vi "ArmLoop2.vi"(11 "ArmRef":T2={"Pot"={"DevStatus"={"status"=FALSE, "code"=0, "source"=""}, "Analog Channel"=enum."Invalid", "Invert Output"=FALSE}, "ArmMotor"={"DeviceStatus"={"status"=FALSE, "code"=0, "source"=""}, "Type"=enum."PWM", "PWM"={"PWM Channel"=enum."Invalid", "DeadBand"={"Name"="", "maxPositivePwm"=0, "minPositivePwm"=0, "centerPwm"=0, "maxNegativePwm"=0, "minNegativePwm"=0, "angularRange"=0}}, "CAN"={"Device Number"=0, "Control Mode"=enum."Percent VBus", "Semaphore"=refnum, "Max Vout"=12.0, "TalonSRX Control Mode"=enum."Percent VBus"}, "Invert"=FALSE}, "Queue"=refnum, "Setpoint"=0.0, "Manual"=FALSE, "output range"={"output high"=100.0, "output low"=-0.38}, "PID gains"={"proportional gain (Kc)"=1.0, "integral time (Ti, min)"=0.01, "derivative time (Td, min)"=0.0}}) -> ()   [LabVIEW 2015, in "ArmController.lvlib"]
uses:
  ArmController.lvlib
  Typedef/ArmRef.ctl
  <vilib>/Rock Robotics/WPI/Potentiometer/WPI_PotentiometerDevRef.ctl
  <vilib>/Rock Robotics/SystemInterfaces/AI/FPGA_AIChannel.ctl
  <vilib>/Rock Robotics/WPI/MotorControl/WPI_MotorControlDeviceRef.ctl
  <vilib>/Rock Robotics/WPI/MotorControl/WPI_MotorControlType.ctl
  <vilib>/Rock Robotics/SystemInterfaces/DIO/FPGA_DIOPWMChannel.ctl
  <vilib>/Rock Robotics/WPI/PWM/WPI_PWMDeadband.ctl
  <vilib>/Rock Robotics/WPI/CAN/Jaguar/SubVIs/WPI_CANJaguar_ControlMode.ctl
  <vilib>/Rock Robotics/WPI/CAN/TalonSRX/WPI_CANTalonSRX_APIControlMode.ctl
  Typedef/MessageType.ctl
  <vilib>/Rock Robotics/Network Tables/NT Write Number.vi
  <vilib>/addons/control/pid/pid.llb/PID Advanced (DBL).vi
  <vilib>/addons/control/pid/NI_PID_pid.lvlib
panel:
  out "Chart":T1(graph)
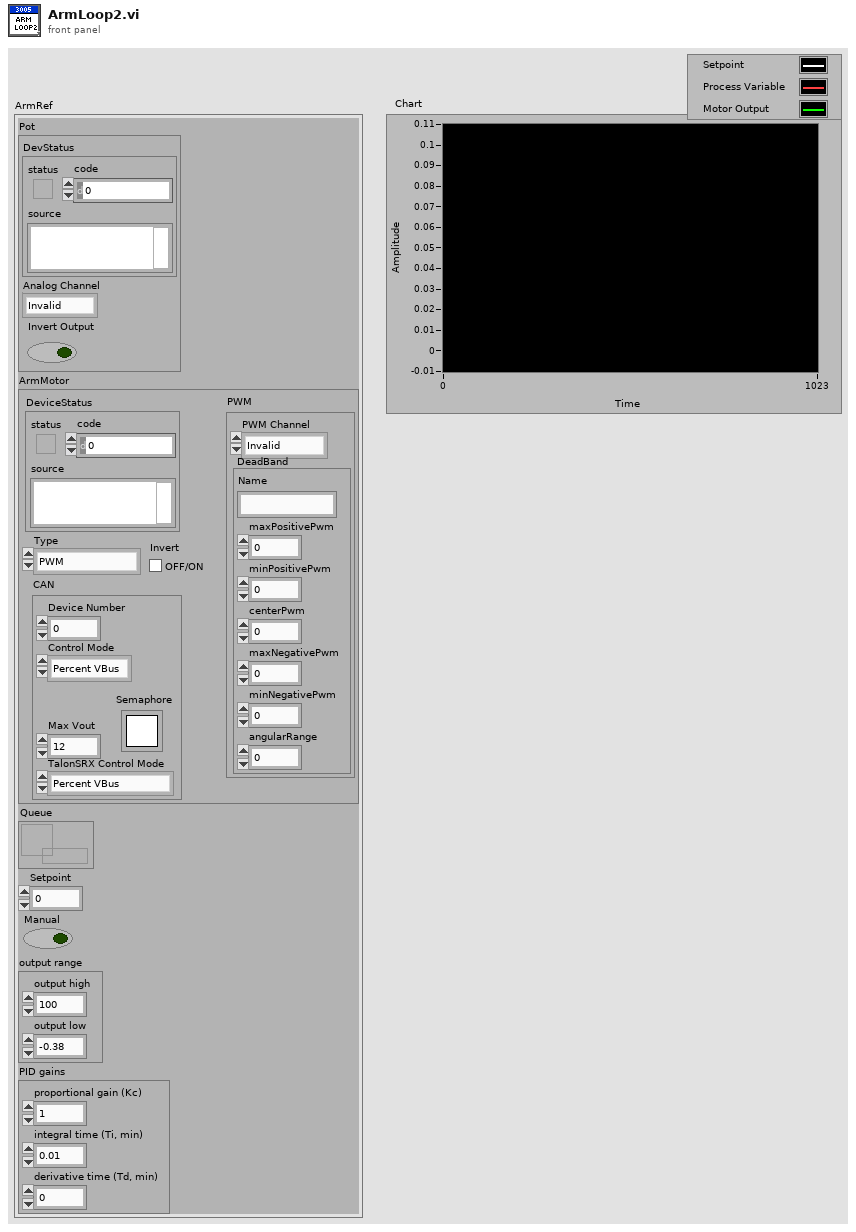
[diagram p1: front panel]
types:
  T1 = cluster{"Value":dbl, "Normalized Value":dbl, "output":dbl}
  T2 = typedef "ArmController.lvlib/ArmRef.ctl" = cluster{"Pot":T3, "ArmMotor":T5, "Queue":refnum<queue>, "Setpoint":dbl, "Manual":bool, "output range":cluster{"output high":dbl, "output low":dbl}, "PID gains":cluster{"proportional gain (Kc)":dbl, "integral time (Ti, min)":dbl, "derivative time (Td, min)":dbl}}
  T3 = typedef "WPI_PotentiometerDevRef.ctl" = cluster{"DevStatus":errorcluster, "Analog Channel":T4, "Invert Output":bool}
  T4 = typedef "FPGA_AIChannel.ctl" = enum8{"AI 0", "AI 1", "AI 2", "AI 3", "AI MXP 0", "AI MXP 1", "AI MXP 2", "AI MXP 3", "Invalid"}
  T5 = typedef "WPI_MotorControlDeviceRef.ctl" = cluster{"DeviceStatus":errorcluster, "Type":T6, "PWM":cluster{"PWM Channel":T7, "DeadBand":T8}, "CAN":cluster{"Device Number":u8, "Control Mode":T9, "Semaphore":T10, "Max Vout":dbl, "TalonSRX Control Mode":T11}, "Invert":bool}
  T6 = typedef "WPI_MotorControlType.ctl" = enum16{"PWM", "CAN", "CANTalonSRX"}
  T7 = typedef "FPGA_DIOPWMChannel.ctl" = enum8{"PWM 0", "PWM 1", "PWM 2", "PWM 3", "PWM 4", "PWM 5", "PWM 6", "PWM 7", "PWM 8", "PWM 9", "PWM MXP 0", "PWM MXP 1", "PWM MXP 2", "PWM MXP 3", "PWM MXP 4", "PWM MXP 5", "PWM MXP 6", "PWM MXP 7", "PWM MXP 8", "PWM MXP 9", "Invalid"}
  T8 = typedef "WPI_PWMDeadband.ctl" = cluster{"Name":string, "maxPositivePwm":i32, "minPositivePwm":i32, "centerPwm":i32, "maxNegativePwm":i32, "minNegativePwm":i32, "angularRange":u16}
  T9 = typedef "WPI_CANJaguar_ControlMode.ctl" = enum8{"Percent VBus", "Current", "Speed", "Position", "Voltage"}
  T10 = typedef "Semaphore RefNum" = refnum<k1>
  T11 = typedef "WPI_CANTalonSRX_APIControlMode.ctl" = enum8{"Percent VBus", "Speed", "Position", "Slave", "Unchanged / Invalid", "Voltage Compensation", "Current", "Motion Profile"}
  T12 = cluster{"proportional gain (Kc)":dbl, "integral time (Ti, min)":dbl, "derivative time (Td, min)":dbl}
  T13 = typedef "ArmController.lvlib/MessageType.ctl" = cluster{"Value":dbl, "Manual Control":bool, "Auto Switch":bool}
  T14 = cluster{"Setpoint":dbl, "Normalized Value":dbl, "output":dbl}
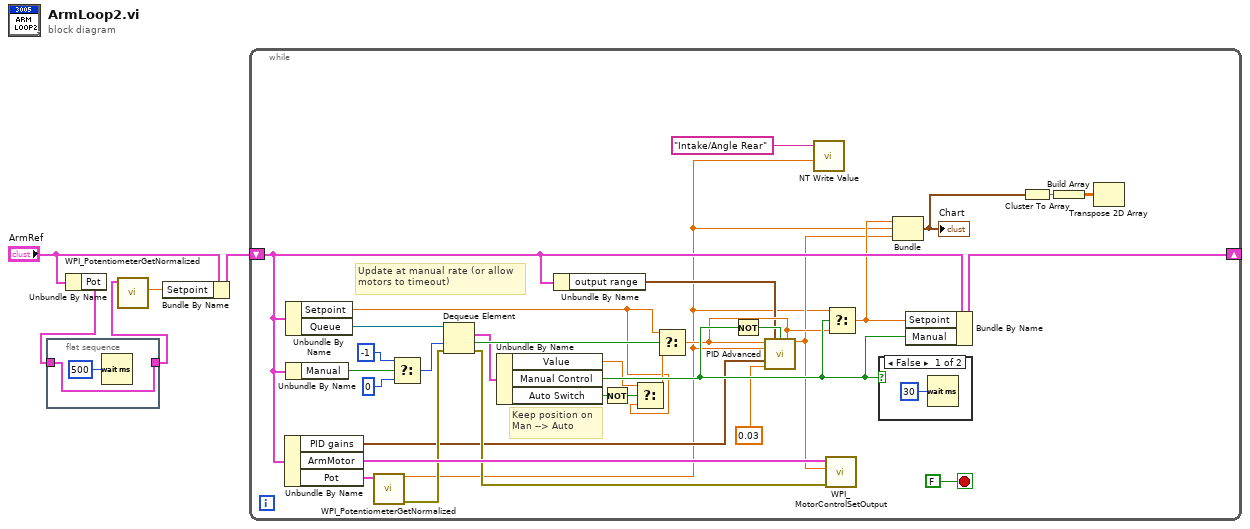
[diagram p0: block diagram]
diagram:
  n1 = flat-sequence {
    tunnel: w2 -> [w6]
    tunnel: [w6] -> w3
    frame #0 {
      n2 = Wait (ms)(milliseconds to wait=u32 500) -> ()  [unwired: 1 out]
    }
  }
  n3 = Unbundle By Name("ArmRef") -> ("Pot"=w2:T3)
  n4 = call <vilib>:"WPI_PotentiometerGetNormalized.vi"("PotDevRef"=w3) -> ("Normalized Value"=w5:dbl)  [unwired: 8 in, 2 out]
  n5 = Bundle By Name(cluster="ArmRef", "Setpoint"=w5) -> (w1:T2)
  n6 = while {
    shift-right: [w35] -> _
    shift-left: w1 -> [w23]
    stop <- FALSE stop-if-true
    # "Keep position on\nMan --> Auto"
    # "Update at manual rate (or allow\nmotors to timeout)"
    n7 = Unbundle By Name(w23) -> ("PID gains"=w18:T12, "ArmMotor"=w34:T5, "Pot"=w36:T3)
    n8 = Unbundle By Name(w23) -> ("Setpoint"=w13:dbl, "Queue"=w39:refnum<queue>)
    n9 = Unbundle By Name(w23) -> ("Manual"=w30:bool)
    n10 = call <vilib>:"WPI_PotentiometerGetNormalized.vi"("PotDevRef"=w36) -> ("error out"=w29:errorcluster, "Normalized Value"=w12:dbl)  [unwired: 8 in, 1 out]
    n11 = Select(t=-1 ("timeout in ms (-1)"), s=w30, f=0 ("timeout in ms (-1)")) -> (s? t:f=w31:i32)
    n12 = Dequeue Element(queue=w39, timeout in ms (-1)=w31, error in (no error)=w29) -> (element=w37:T13, timed out?=w38:bool, error out=w28:errorcluster)  [unwired: 1 out]
    n13 = Unbundle By Name(w37) -> ("Value"=w15:dbl, "Manual Control"=w27:bool, "Auto Switch"=w17:bool)
    n14 = Unbundle By Name(w23) -> ("output range"=w19:cluster{"output high":dbl, "output low":dbl})
    n15 = Not(x=w17) -> (.not. x?=w14:bool)
    n16 = Select(t=w15, s=w14, f=w13) -> (s? t:f=w16:dbl)
    n17 = Select(t=w13, s=w38, f=w16) -> (s? t:f=w26:dbl)
    n18 = Not(x=w27) -> (.not. x?=w20:bool)
    n19 = call-poly <vilib>:"PID Advanced.vi"("setpoint"=w26, "output range"=w19, "auto? (T)"=w20, "manual control"=w26, "process variable"=w12, "PID gains"=w18, "dt (s)"=0.03) -> ("output"=w21:dbl)  [unwired: 7 in, 1 out]
    n20 = call-poly <vilib>:"NT Write Value.vi"("Numeric"=w12, "Name"="Intake/Angle Rear") -> ()  [unwired: 9 in, 1 out]
    n21 = call <vilib>:"WPI_MotorControlSetOutput.vi"("error in (no error)"=w28, "Output"=w21, "MotorControlDevRef"=w34) -> ()  [unwired: 6 in, 3 out]
    n22 = Select(t=w12, s=w27, f=w26) -> (s? t:f=w22:dbl)
    n23 = case shown="False" w27 {
      frame False {
        n24 = Wait (ms)(milliseconds to wait=u32 30) -> ()  [unwired: 1 out]
      }
      frame True {
      }
    }
    n25 = Bundle("Setpoint"=w22, "Normalized Value"=w12, "output"=w21) -> (w8:T14)  [unwired: 1 in]
    "Chart" <- w8
    n26 = Bundle By Name(cluster=w23, "Setpoint"=w22, "Manual"=w27) -> (w35:T2)
    n27 = Cluster To Array(cluster=w8) -> (array=w10:dbl[])
    n28 = Build Array(w10) -> (w9:dbl[][])
    n29 = Transpose 2D Array(2D array=w9) -> ()  [unwired: 1 out]
  }
